vi "Initialize.vi"(7 "ChannelName":string="Setpoint.ch%d.SP", 8 "error in":errorcluster, 9 "Number of Channels":u32=1, 10 "Instance Name":string, 11 "Actual Value in":refnum<class "Actual Value.lvclass">) -> (0 "error out":errorcluster, 3 "Actual Value out":refnum<class "Actual Value.lvclass">)   [LabVIEW 2023, in "Actual Value.lvclass"]
uses:
  Actual Value.lvclass
  Actual Value.lvclass/Actual Value.ctl
  bls-capabilities/src/Capabilities/Utilities/Utilities.lvlib
  <vilib>/ADAS Replay HIL/Channels/Tag Wrapper/Tag Wrapper.lvlib
  <vilib>/ADAS Replay HIL/Channels/Tag Wrapper/Polymorphic/Set Default Value (Double).vi
  <vilib>/ADAS Replay HIL/Channels/Tag Wrapper/Polymorphic/Open Producer Tag (Double).vi
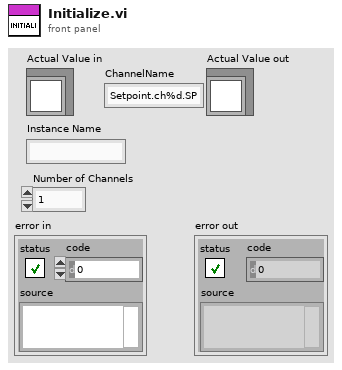
[diagram p1: front panel]
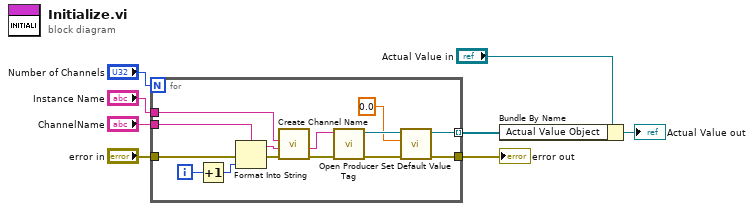
[diagram p0: block diagram]
diagram:
  n1 = for {
    N: "Number of Channels" -> [_]
    tunnel: [w10] -> w2 mode=indexing
    tunnel: [w9] -> w5
    tunnel: "ChannelName" -> [w20]
    tunnel: "Instance Name" -> [w22]
    tunnel: "error in" -> [w16]
    i -> [w19]
    n2 = Increment(x=w19) -> (x+1=w18:i32)
    n3 = Format Into String(format string=w20, error in=w16, w18) -> (resulting string=w21:string, error out=w17:errorcluster)  [unwired: 1 in]
    n4 = call "Create Channel Name.vi"("error in"=w17, "Channel Name"=w21, "Plugin Name"=w22) -> ("error out"=w12:errorcluster, "Data Channel Name"=w11:string)  [unwired: 7 in]
    n5 = call-poly <vilib>:"Open Producer Tag.vi"("error in"=w12, "Channel Name"=w11) -> ("error out"=w15:errorcluster, "ADAS HIL Channel"=w14:refnum<k21>)  [unwired: 8 in]
    n6 = call-poly <vilib>:"Set Default Value.vi"("error in"=w15, "Default Value"=0.0, "ADAS HIL Channel in"=w14) -> ("error out"=w9:errorcluster, "ADAS HIL Channel out"=w10:refnum<k21>)  [unwired: 7 in]
  }
  "error out" <- w5
  n7 = Bundle By Name(cluster="Actual Value in", "Actual Value Object"=w2) -> (→"Actual Value out":refnum<class "Actual Value.lvclass">)
